vi "I(V) at various fields_K6221-K2182A_PK.vi"() -> ()   [LabVIEW 2016]
uses:
  Labview Drivers/Keithley 622x LV 2009/Keithley 622x.lvlib
panel:
  in  "Numeric Average":i32=50
  out "Iset (A)":dbl=-4.3999999999999985e-06
  out "data":dbl[](array[numeric])=[-1.0767123e-06, -4.299999999999999e-06, 0.25039820930232565]
  out "I vs V":cluster{dbl, "Field Reading":dbl}[](graph)=[{-2.65213861e-07, "Field Reading"=0.0}, {-2.06331562e-07, "Field Reading"=1e-07}, {-2.45753416e-07, "Field Reading"=2e-07}, {-2.41658661e-07, "Field Reading"=3e-07}, {-2.45242211e-07, "Field Reading"=4e-07}, {-2.44727893e-07, "Field Reading"=5e-07}, {-1.955806e-07, "Field Reading"=6e-07}, {-2.17089385e-07, "Field Reading"=7e-07}, {-2.81598074e-07, "Field Reading"=8e-07}, {-2.74937155e-07, "Field Reading"=9e-07}, {-2.57527922e-07, "Field Reading"=1e-06}, {-1.97112335e-07, "Field Reading"=1.1e-06}, {-1.8175889e-07, "Field Reading"=1.2e-06}, {-2.14527365e-07, "Field Reading"=1.2999999999999998e-06}, {-1.61276589e-07, "Field Reading"=1.3999999999999997e-06}, {-5.88852258e-08, "Field Reading"=1.4999999999999996e-06}, {4.14620688e-08, "Field Reading"=1.5999999999999995e-06}, {4.55608442e-08, "Field Reading"=1.6999999999999994e-06}, {1.10074806e-07, "Field Reading"=1.7999999999999993e-06}, {9.16432587e-08, "Field Reading"=1.8999999999999992e-06}, {2.22710882e-07, "Field Reading"=1.999999999999999e-06}, {2.90806804e-07, "Field Reading"=2.099999999999999e-06}, {2.74933923e-07, "Field Reading"=2.199999999999999e-06}, {2.81079697e-07, "Field Reading"=2.2999999999999987e-06}, {3.16914884e-07, "Field Reading"=2.3999999999999986e-06}, {2.95409204e-07, "Field Reading"=2.4999999999999985e-06}, {3.58898183e-07, "Field Reading"=2.5999999999999984e-06}, {3.56848457e-07, "Field Reading"=2.6999999999999983e-06}, {4.40815949e-07, "Field Reading"=2.799999999999998e-06}, {4.45430022e-07, "Field Reading"=2.899999999999998e-06}, {4.50042171e-07, "Field Reading"=2.999999999999998e-06}, {5.23763566e-07, "Field Reading"=3.099999999999998e-06}, {5.54477469e-07, "Field Reading"=3.1999999999999977e-06}, {5.89806137e-07, "Field Reading"=3.2999999999999976e-06}, {6.03627656e-07, "Field Reading"=3.3999999999999975e-06}, {6.54317135e-07, "Field Reading"=3.4999999999999974e-06}, {7.12174301e-07, "Field Reading"=3.5999999999999973e-06}, {7.36747564e-07, "Field Reading"=3.699999999999997e-06}, {8.03819501e-07, "Field Reading"=3.799999999999997e-06}, {8.68836656e-07, "Field Reading"=3.899999999999997e-06}, {9.59970204e-07, "Field Reading"=3.999999999999997e-06}, {9.96323249e-07, "Field Reading"=4.099999999999997e-06}, {1.07823925e-06, "Field Reading"=4.199999999999997e-06}, {1.11458965e-06, "Field Reading"=4.299999999999997e-06}, {1.11817613e-06, "Field Reading"=4.399999999999997e-06}, {1.23695717e-06, "Field Reading"=4.499999999999997e-06}, {1.24360737e-06, "Field Reading"=4.599999999999997e-06}, {1.27996158e-06, "Field Reading"=4.6999999999999965e-06}, {1.30914358e-06, "Field Reading"=4.799999999999996e-06}, {1.29941092e-06, "Field Reading"=4.899999999999996e-06}, {1.45659309e-06, "Field Reading"=4.999999999999996e-06}, {1.47759059e-06, "Field Reading"=5.099999999999996e-06}, {1.56462638e-06, "Field Reading"=5.199999999999996e-06}, {1.56923247e-06, "Field Reading"=5.299999999999996e-06}, {1.5958572e-06, "Field Reading"=5.399999999999996e-06}, {1.62196573e-06, "Field Reading"=5.499999999999996e-06}, {1.65985372e-06, "Field Reading"=5.5999999999999955e-06}, {1.66548618e-06, "Field Reading"=5.699999999999995e-06}, {1.73869841e-06, "Field Reading"=5.799999999999995e-06}, {1.75918207e-06, "Field Reading"=5.899999999999995e-06}, {1.82420779e-06, "Field Reading"=5.999999999999995e-06}, {1.87539735e-06, "Field Reading"=6.099999999999995e-06}, {2.02541342e-06, "Field Reading"=6.199999999999995e-06}, {2.05920615e-06, "Field Reading"=6.299999999999995e-06}, {2.0607414e-06, "Field Reading"=6.399999999999995e-06}, {2.09299708e-06, "Field Reading"=6.4999999999999945e-06}, {2.14470835e-06, "Field Reading"=6.599999999999994e-06}, {2.22560209e-06, "Field Reading"=6.699999999999994e-06}, {2.29164603e-06, "Field Reading"=6.799999999999994e-06}, {2.29522927e-06, "Field Reading"=6.899999999999994e-06}, {2.34898799e-06, "Field Reading"=6.999999999999994e-06}, {2.35974308e-06, "Field Reading"=7.099999999999994e-06}, {2.33516555e-06, "Field Reading"=7.199999999999994e-06}, {2.38277613e-06, "Field Reading"=7.299999999999994e-06}, {2.52971809e-06, "Field Reading"=7.3999999999999935e-06}, {2.52562488e-06, "Field Reading"=7.499999999999993e-06}, {2.53073687e-06, "Field Reading"=7.599999999999993e-06}, {2.67562896e-06, "Field Reading"=7.699999999999994e-06}, {2.75038341e-06, "Field Reading"=7.799999999999995e-06}, {2.77444721e-06, "Field Reading"=7.899999999999996e-06}, {2.86045666e-06, "Field Reading"=7.999999999999996e-06}, {2.95312204e-06, "Field Reading"=8.099999999999997e-06}, {2.99612267e-06, "Field Reading"=8.199999999999998e-06}, {2.98793425e-06, "Field Reading"=8.299999999999998e-06}, {3.08214364e-06, "Field Reading"=8.4e-06}, {3.07036496e-06, "Field Reading"=8.5e-06}, {3.17481336e-06, "Field Reading"=8.6e-06}, {3.13692748e-06, "Field Reading"=8.700000000000001e-06}, {3.13795104e-06, "Field Reading"=8.800000000000002e-06}, {3.21679593e-06, "Field Reading"=8.900000000000003e-06}, {3.24444364e-06, "Field Reading"=9.000000000000004e-06}, {3.34223395e-06, "Field Reading"=9.100000000000004e-06}, {3.37244308e-06, "Field Reading"=9.200000000000005e-06}, {3.49890549e-06, "Field Reading"=9.300000000000006e-06}, {3.5705844e-06, "Field Reading"=9.400000000000007e-06}, {3.56136e-06, "Field Reading"=9.500000000000007e-06}, {3.64941777e-06, "Field Reading"=9.600000000000008e-06}, {3.65403077e-06, "Field Reading"=9.700000000000009e-06}, {3.70881304e-06, "Field Reading"=9.80000000000001e-06}, {3.74413912e-06, "Field Reading"=9.90000000000001e-06}, {3.78202672e-06, "Field Reading"=1.0000000000000011e-05}, {3.77588359e-06, "Field Reading"=1.0100000000000012e-05}, {3.79482737e-06, "Field Reading"=1.0200000000000012e-05}, {3.84807257e-06, "Field Reading"=1.0300000000000013e-05}, {3.96326851e-06, "Field Reading"=1.0400000000000014e-05}, {4.02675375e-06, "Field Reading"=1.0500000000000015e-05}, {4.01548692e-06, "Field Reading"=1.0600000000000015e-05}, {4.03188336e-06, "Field Reading"=1.0700000000000016e-05}, {4.11892625e-06, "Field Reading"=1.0800000000000017e-05}, {4.16499723e-06, "Field Reading"=1.0900000000000018e-05}, {4.13786622e-06, "Field Reading"=1.1000000000000018e-05}, {4.15936464e-06, "Field Reading"=1.1100000000000019e-05}, {4.15372248e-06, "Field Reading"=1.120000000000002e-05}, {4.1921208e-06, "Field Reading"=1.130000000000002e-05}, {4.20441259e-06, "Field Reading"=1.1400000000000021e-05}, {4.22285166e-06, "Field Reading"=1.1500000000000022e-05}, {4.41023425e-06, "Field Reading"=1.1600000000000023e-05}, {4.43121181e-06, "Field Reading"=1.1700000000000024e-05}, {4.48548487e-06, "Field Reading"=1.1800000000000024e-05}, {4.51827063e-06, "Field Reading"=1.1900000000000025e-05}, {4.56332253e-06, "Field Reading"=1.2000000000000026e-05}, {4.56996768e-06, "Field Reading"=1.2100000000000026e-05}, {4.61196138e-06, "Field Reading"=1.2200000000000027e-05}, {4.66060156e-06, "Field Reading"=1.2300000000000028e-05}, {4.71282017e-06, "Field Reading"=1.2400000000000029e-05}, {4.72562207e-06, "Field Reading"=1.250000000000003e-05}, {4.80549203e-06, "Field Reading"=1.260000000000003e-05}, {4.84132842e-06, "Field Reading"=1.2700000000000031e-05}, {4.81931379e-06, "Field Reading"=1.2800000000000032e-05}, {4.91812376e-06, "Field Reading"=1.2900000000000032e-05}, {4.97443564e-06, "Field Reading"=1.3000000000000033e-05}, {5.06864178e-06, "Field Reading"=1.3100000000000034e-05}, {5.15414621e-06, "Field Reading"=1.3200000000000035e-05}, {5.14594912e-06, "Field Reading"=1.3300000000000035e-05}, {5.15516684e-06, "Field Reading"=1.3400000000000036e-05}, {5.24221524e-06, "Field Reading"=1.3500000000000037e-05}, {5.29853469e-06, "Field Reading"=1.3600000000000038e-05}, {5.35638168e-06, "Field Reading"=1.3700000000000038e-05}, {5.37020179e-06, "Field Reading"=1.3800000000000039e-05}, {5.3492118e-06, "Field Reading"=1.390000000000004e-05}, {5.39375972e-06, "Field Reading"=1.400000000000004e-05}, {5.47056068e-06, "Field Reading"=1.4100000000000041e-05}, {5.50895206e-06, "Field Reading"=1.4200000000000042e-05}, {5.5514459e-06, "Field Reading"=1.4300000000000043e-05}, {5.55707986e-06, "Field Reading"=1.4400000000000043e-05}, {5.60366331e-06, "Field Reading"=1.4500000000000044e-05}, {5.64206701e-06, "Field Reading"=1.4600000000000045e-05}, {5.75061982e-06, "Field Reading"=1.4700000000000046e-05}, {5.78440485e-06, "Field Reading"=1.4800000000000046e-05}, {5.84225116e-06, "Field Reading"=1.4900000000000047e-05}, {5.85863506e-06, "Field Reading"=1.5000000000000048e-05}, {5.91290279e-06, "Field Reading"=1.5100000000000049e-05}, {5.90009794e-06, "Field Reading"=1.520000000000005e-05}, {5.99225908e-06, "Field Reading"=1.530000000000005e-05}, {6.0357811e-06, "Field Reading"=1.540000000000005e-05}, {6.09005686e-06, "Field Reading"=1.5500000000000048e-05}, {6.16276569e-06, "Field Reading"=1.5600000000000047e-05}, {6.223172e-06, "Field Reading"=1.5700000000000046e-05}, {6.27077906e-06, "Field Reading"=1.5800000000000045e-05}, {6.31429835e-06, "Field Reading"=1.5900000000000044e-05}, {6.34911719e-06, "Field Reading"=1.6000000000000043e-05}, {6.38342782e-06, "Field Reading"=1.6100000000000042e-05}, {6.40851838e-06, "Field Reading"=1.620000000000004e-05}, {6.46738862e-06, "Field Reading"=1.630000000000004e-05}, {6.49911838e-06, "Field Reading"=1.640000000000004e-05}, {6.55799613e-06, "Field Reading"=1.650000000000004e-05}, {6.62046237e-06, "Field Reading"=1.6600000000000038e-05}, {6.63786331e-06, "Field Reading"=1.6700000000000037e-05}, {6.73360462e-06, "Field Reading"=1.6800000000000036e-05}, {6.76740248e-06, "Field Reading"=1.6900000000000035e-05}, {6.79761286e-06, "Field Reading"=1.7000000000000034e-05}, {6.87696878e-06, "Field Reading"=1.7100000000000033e-05}, {6.92663472e-06, "Field Reading"=1.7200000000000032e-05}, {6.96504415e-06, "Field Reading"=1.730000000000003e-05}, {7.05310834e-06, "Field Reading"=1.740000000000003e-05}, {7.1360323e-06, "Field Reading"=1.750000000000003e-05}, {7.18210114e-06, "Field Reading"=1.7600000000000028e-05}, {7.20208147e-06, "Field Reading"=1.7700000000000027e-05}, {7.28861423e-06, "Field Reading"=1.7800000000000026e-05}, {7.33519871e-06, "Field Reading"=1.7900000000000025e-05}, {7.44937016e-06, "Field Reading"=1.8000000000000024e-05}, {7.48215567e-06, "Field Reading"=1.8100000000000023e-05}, {7.55229248e-06, "Field Reading"=1.8200000000000022e-05}, {7.5732755e-06, "Field Reading"=1.830000000000002e-05}, {7.68847322e-06, "Field Reading"=1.840000000000002e-05}, {7.65775525e-06, "Field Reading"=1.850000000000002e-05}, {7.67208615e-06, "Field Reading"=1.860000000000002e-05}, {7.7637263e-06, "Field Reading"=1.8700000000000017e-05}, {7.84923772e-06, "Field Reading"=1.8800000000000017e-05}, {7.85384559e-06, "Field Reading"=1.8900000000000016e-05}, {7.90913653e-06, "Field Reading"=1.9000000000000015e-05}, {7.93422015e-06, "Field Reading"=1.9100000000000014e-05}, {8.02791857e-06, "Field Reading"=1.9200000000000013e-05}, {8.06375894e-06, "Field Reading"=1.9300000000000012e-05}, {8.08936091e-06, "Field Reading"=1.940000000000001e-05}, {8.13646665e-06, "Field Reading"=1.950000000000001e-05}, {8.17230556e-06, "Field Reading"=1.960000000000001e-05}, {8.25165814e-06, "Field Reading"=1.9700000000000008e-05}, {8.28083444e-06, "Field Reading"=1.9800000000000007e-05}, {8.32742883e-06, "Field Reading"=1.9900000000000006e-05}, {8.40371126e-06, "Field Reading"=2e-05}, {8.32588703e-06, "Field Reading"=1.9900000000000003e-05}, {8.27059152e-06, "Field Reading"=1.9800000000000004e-05}, {8.24550498e-06, "Field Reading"=1.9700000000000005e-05}, {8.18766651e-06, "Field Reading"=1.9600000000000005e-05}, {8.16002117e-06, "Field Reading"=1.9500000000000006e-05}, {8.11034423e-06, "Field Reading"=1.9400000000000007e-05}, {8.06631431e-06, "Field Reading"=1.930000000000001e-05}, {7.96853626e-06, "Field Reading"=1.920000000000001e-05}, {7.96494837e-06, "Field Reading"=1.910000000000001e-05}, {7.88456389e-06, "Field Reading"=1.900000000000001e-05}, {7.84667228e-06, "Field Reading"=1.8900000000000012e-05}, {7.76577688e-06, "Field Reading"=1.8800000000000013e-05}, {7.72174608e-06, "Field Reading"=1.8700000000000014e-05}, {7.70996248e-06, "Field Reading"=1.8600000000000015e-05}, {7.64032909e-06, "Field Reading"=1.8500000000000016e-05}, {7.58196852e-06, "Field Reading"=1.8400000000000017e-05}, {7.52616124e-06, "Field Reading"=1.8300000000000018e-05}, {7.43451656e-06, "Field Reading"=1.820000000000002e-05}, {7.419165e-06, "Field Reading"=1.810000000000002e-05}, {7.41302153e-06, "Field Reading"=1.800000000000002e-05}, {7.40278217e-06, "Field Reading"=1.7900000000000022e-05}, {7.34748378e-06, "Field Reading"=1.7800000000000023e-05}, {7.26146266e-06, "Field Reading"=1.7700000000000024e-05}, {7.22614421e-06, "Field Reading"=1.7600000000000025e-05}, {7.15294258e-06, "Field Reading"=1.7500000000000026e-05}, {7.13912167e-06, "Field Reading"=1.7400000000000027e-05}, {7.05105581e-06, "Field Reading"=1.7300000000000027e-05}, {7.06896784e-06, "Field Reading"=1.720000000000003e-05}, {6.98551895e-06, "Field Reading"=1.710000000000003e-05}, {6.92254427e-06, "Field Reading"=1.700000000000003e-05}, {6.86724585e-06, "Field Reading"=1.690000000000003e-05}, {6.85240011e-06, "Field Reading"=1.6800000000000032e-05}, {6.78225464e-06, "Field Reading"=1.6700000000000033e-05}, {6.77713724e-06, "Field Reading"=1.6600000000000034e-05}, {6.69368315e-06, "Field Reading"=1.6500000000000035e-05}, {6.63224313e-06, "Field Reading"=1.6400000000000036e-05}, {6.64145914e-06, "Field Reading"=1.6300000000000037e-05}, {6.55391401e-06, "Field Reading"=1.6200000000000038e-05}, {6.54776972e-06, "Field Reading"=1.610000000000004e-05}, {6.44434302e-06, "Field Reading"=1.600000000000004e-05}, {6.37830276e-06, "Field Reading"=1.590000000000004e-05}, {6.32249712e-06, "Field Reading"=1.5800000000000042e-05}, {6.30507964e-06, "Field Reading"=1.5700000000000043e-05}, {6.27589889e-06, "Field Reading"=1.5600000000000044e-05}, {6.19193872e-06, "Field Reading"=1.5500000000000045e-05}, {6.14893632e-06, "Field Reading"=1.5400000000000046e-05}, {6.10695312e-06, "Field Reading"=1.5300000000000047e-05}, {6.07315478e-06, "Field Reading"=1.5200000000000046e-05}, {6.01376066e-06, "Field Reading"=1.5100000000000045e-05}, {6.01273927e-06, "Field Reading"=1.5000000000000044e-05}, {5.94362298e-06, "Field Reading"=1.4900000000000044e-05}, {5.89037156e-06, "Field Reading"=1.4800000000000043e-05}, {5.87757219e-06, "Field Reading"=1.4700000000000042e-05}, {5.83406487e-06, "Field Reading"=1.4600000000000041e-05}, {5.7818526e-06, "Field Reading"=1.450000000000004e-05}, {5.79054303e-06, "Field Reading"=1.440000000000004e-05}, {5.72397236e-06, "Field Reading"=1.430000000000004e-05}, {5.69632955e-06, "Field Reading"=1.4200000000000039e-05}, {5.62875043e-06, "Field Reading"=1.4100000000000038e-05}, {5.61902647e-06, "Field Reading"=1.4000000000000037e-05}, {5.53097021e-06, "Field Reading"=1.3900000000000036e-05}, {5.58626586e-06, "Field Reading"=1.3800000000000036e-05}, {5.5396681e-06, "Field Reading"=1.3700000000000035e-05}, {5.49102684e-06, "Field Reading"=1.3600000000000034e-05}, {5.46030697e-06, "Field Reading"=1.3500000000000033e-05}, {5.39784099e-06, "Field Reading"=1.3400000000000033e-05}, {5.28981952e-06, "Field Reading"=1.3300000000000032e-05}, {5.3456268e-06, "Field Reading"=1.3200000000000031e-05}, {5.23811359e-06, "Field Reading"=1.310000000000003e-05}, {5.28317073e-06, "Field Reading"=1.300000000000003e-05}, {5.23554661e-06, "Field Reading"=1.2900000000000029e-05}, {5.18742312e-06, "Field Reading"=1.2800000000000028e-05}, {5.16080263e-06, "Field Reading"=1.2700000000000027e-05}, {5.08911473e-06, "Field Reading"=1.2600000000000027e-05}, {5.02306725e-06, "Field Reading"=1.2500000000000026e-05}, {4.95087495e-06, "Field Reading"=1.2400000000000025e-05}, {4.89097002e-06, "Field Reading"=1.2300000000000025e-05}, {4.85103666e-06, "Field Reading"=1.2200000000000024e-05}, {4.81161312e-06, "Field Reading"=1.2100000000000023e-05}, {4.8223712e-06, "Field Reading"=1.2000000000000022e-05}, {4.71997748e-06, "Field Reading"=1.1900000000000022e-05}, {4.70513009e-06, "Field Reading"=1.1800000000000021e-05}, {4.61860758e-06, "Field Reading"=1.170000000000002e-05}, {4.50494221e-06, "Field Reading"=1.160000000000002e-05}, {4.50442328e-06, "Field Reading"=1.1500000000000019e-05}, {4.48907395e-06, "Field Reading"=1.1400000000000018e-05}, {4.48549552e-06, "Field Reading"=1.1300000000000017e-05}, {4.43275985e-06, "Field Reading"=1.1200000000000016e-05}, {4.37336829e-06, "Field Reading"=1.1100000000000016e-05}, {4.35544798e-06, "Field Reading"=1.1000000000000015e-05}, {4.23615778e-06, "Field Reading"=1.0900000000000014e-05}, {4.18496019e-06, "Field Reading"=1.0800000000000013e-05}, {4.13529928e-06, "Field Reading"=1.0700000000000013e-05}, {4.0963864e-06, "Field Reading"=1.0600000000000012e-05}, {4.10252432e-06, "Field Reading"=1.0500000000000011e-05}, {4.14245452e-06, "Field Reading"=1.040000000000001e-05}, {4.0723185e-06, "Field Reading"=1.030000000000001e-05}, {3.99655577e-06, "Field Reading"=1.0200000000000009e-05}, {3.91820595e-06, "Field Reading"=1.0100000000000008e-05}, {3.90693848e-06, "Field Reading"=1.0000000000000008e-05}, {3.90182893e-06, "Field Reading"=9.900000000000007e-06}, {3.89824771e-06, "Field Reading"=9.800000000000006e-06}, {3.89568225e-06, "Field Reading"=9.700000000000005e-06}, {3.82297919e-06, "Field Reading"=9.600000000000005e-06}, {3.79072008e-06, "Field Reading"=9.500000000000004e-06}, {3.75283128e-06, "Field Reading"=9.400000000000003e-06}, {3.74925146e-06, "Field Reading"=9.300000000000002e-06}, {3.69600662e-06, "Field Reading"=9.200000000000002e-06}, {3.68985764e-06, "Field Reading"=9.100000000000001e-06}, {3.53830951e-06, "Field Reading"=9e-06}, {3.48967903e-06, "Field Reading"=8.9e-06}, {3.4169754e-06, "Field Reading"=8.799999999999999e-06}, {3.35195893e-06, "Field Reading"=8.699999999999998e-06}, {3.26798993e-06, "Field Reading"=8.599999999999997e-06}, {3.32840376e-06, "Field Reading"=8.499999999999997e-06}, {3.28130617e-06, "Field Reading"=8.399999999999996e-06}, {3.22038204e-06, "Field Reading"=8.299999999999995e-06}, {3.19170899e-06, "Field Reading"=8.199999999999994e-06}, {3.14817946e-06, "Field Reading"=8.099999999999994e-06}, {3.06473437e-06, "Field Reading"=7.999999999999993e-06}, {3.0155901e-06, "Field Reading"=7.899999999999992e-06}, {2.89219787e-06, "Field Reading"=7.799999999999991e-06}, {2.84355222e-06, "Field Reading"=7.69999999999999e-06}, {2.79798017e-06, "Field Reading"=7.599999999999991e-06}, {2.73245105e-06, "Field Reading"=7.499999999999991e-06}, {2.68023355e-06, "Field Reading"=7.399999999999991e-06}, {2.76420187e-06, "Field Reading"=7.299999999999991e-06}, {2.74935814e-06, "Field Reading"=7.199999999999991e-06}, {2.68791939e-06, "Field Reading"=7.099999999999991e-06}, {2.63261821e-06, "Field Reading"=6.9999999999999914e-06}, {2.60291933e-06, "Field Reading"=6.8999999999999915e-06}, {2.51843848e-06, "Field Reading"=6.799999999999992e-06}, {2.5061508e-06, "Field Reading"=6.699999999999992e-06}, {2.33208474e-06, "Field Reading"=6.599999999999992e-06}, {2.3167298e-06, "Field Reading"=6.499999999999992e-06}, {2.30443977e-06, "Field Reading"=6.399999999999992e-06}, {2.24402212e-06, "Field Reading"=6.299999999999992e-06}, {2.26142112e-06, "Field Reading"=6.199999999999992e-06}, {2.24708744e-06, "Field Reading"=6.099999999999992e-06}, {2.18258492e-06, "Field Reading"=5.9999999999999925e-06}, {2.06226311e-06, "Field Reading"=5.899999999999993e-06}, {1.97317707e-06, "Field Reading"=5.799999999999993e-06}, {1.89791536e-06, "Field Reading"=5.699999999999993e-06}, {1.8943317e-06, "Field Reading"=5.599999999999993e-06}, {1.91123261e-06, "Field Reading"=5.499999999999993e-06}, {1.79142144e-06, "Field Reading"=5.399999999999993e-06}, {1.82674468e-06, "Field Reading"=5.299999999999993e-06}, {1.75353415e-06, "Field Reading"=5.199999999999993e-06}, {1.65932968e-06, "Field Reading"=5.0999999999999935e-06}, {1.65933232e-06, "Field Reading"=4.999999999999994e-06}, {1.54669792e-06, "Field Reading"=4.899999999999994e-06}, {1.44584143e-06, "Field Reading"=4.799999999999994e-06}, {1.52673386e-06, "Field Reading"=4.699999999999994e-06}, {1.4320141e-06, "Field Reading"=4.599999999999994e-06}, {1.40795279e-06, "Field Reading"=4.499999999999994e-06}, {1.32296227e-06, "Field Reading"=4.399999999999994e-06}, {1.08181445e-06, "Field Reading"=4.299999999999994e-06}, {1.07105849e-06, "Field Reading"=4.1999999999999945e-06}, {1.07361536e-06, "Field Reading"=4.099999999999995e-06}, {1.06030613e-06, "Field Reading"=3.999999999999995e-06}, {9.90675451e-07, "Field Reading"=3.899999999999995e-06}, {9.98353274e-07, "Field Reading"=3.799999999999995e-06}, {9.51769766e-07, "Field Reading"=3.699999999999995e-06}, {9.19007087e-07, "Field Reading"=3.599999999999995e-06}, {8.96477356e-07, "Field Reading"=3.4999999999999953e-06}, {8.37598555e-07, "Field Reading"=3.3999999999999954e-06}, {7.43906148e-07, "Field Reading"=3.2999999999999955e-06}, {7.07042824e-07, "Field Reading"=3.1999999999999956e-06}, {7.8384287e-07, "Field Reading"=3.0999999999999957e-06}, {6.97316697e-07, "Field Reading"=2.999999999999996e-06}, {6.99871857e-07, "Field Reading"=2.899999999999996e-06}, {6.61988855e-07, "Field Reading"=2.799999999999996e-06}, {6.67112949e-07, "Field Reading"=2.699999999999996e-06}, {5.21710306e-07, "Field Reading"=2.5999999999999963e-06}, {5.11980802e-07, "Field Reading"=2.4999999999999964e-06}, {5.26306067e-07, "Field Reading"=2.3999999999999965e-06}, {5.57538796e-07, "Field Reading"=2.2999999999999966e-06}, {5.49862592e-07, "Field Reading"=2.1999999999999967e-06}, {4.38246539e-07, "Field Reading"=2.099999999999997e-06}, {4.53099149e-07, "Field Reading"=1.999999999999997e-06}, {3.79374306e-07, "Field Reading"=1.899999999999997e-06}, {3.25102595e-07, "Field Reading"=1.7999999999999972e-06}, {2.04792301e-07, "Field Reading"=1.6999999999999973e-06}, {2.36019239e-07, "Field Reading"=1.5999999999999974e-06}, {2.33452923e-07, "Field Reading"=1.4999999999999975e-06}, {2.2372704e-07, "Field Reading"=1.3999999999999976e-06}, {2.67761542e-07, "Field Reading"=1.2999999999999977e-06}, {2.54450874e-07, "Field Reading"=1.1999999999999978e-06}, {1.63316468e-07, "Field Reading"=1.099999999999998e-06}, {7.72994096e-08, "Field Reading"=9.99999999999998e-07}, {8.85529671e-08, "Field Reading"=8.999999999999981e-07}, {7.06354729e-08, "Field Reading"=7.999999999999981e-07}, {1.87884609e-07, "Field Reading"=6.999999999999981e-07}, {1.58696118e-07, "Field Reading"=5.999999999999981e-07}, {1.73034013e-07, "Field Reading"=4.999999999999981e-07}, {1.02383086e-07, "Field Reading"=3.999999999999981e-07}, {6.60310964e-08, "Field Reading"=2.999999999999981e-07}, {1.43341752e-07, "Field Reading"=1.9999999999999809e-07}, {2.34987166e-07, "Field Reading"=9.999999999999809e-08}, {1.56651714e-07, "Field Reading"=-1.9058241313221758e-21}, {1.5204492e-07, "Field Reading"=-1.000000000000019e-07}, {2.03758966e-07, "Field Reading"=-2.000000000000019e-07}, {2.2474776e-07, "Field Reading"=-3.000000000000019e-07}, {1.65354644e-07, "Field Reading"=-4.000000000000019e-07}, {1.18764208e-07, "Field Reading"=-5.000000000000019e-07}, {7.88302354e-08, "Field Reading"=-6.000000000000019e-07}, {1.93518827e-07, "Field Reading"=-7.000000000000019e-07}, {1.5665572e-07, "Field Reading"=-8.000000000000019e-07}, {2.47273023e-07, "Field Reading"=-9.000000000000019e-07}, {2.08356789e-07, "Field Reading"=-1.0000000000000019e-06}, {2.10917939e-07, "Field Reading"=-1.1000000000000018e-06}, {1.69965974e-07, "Field Reading"=-1.2000000000000016e-06}, {1.11596254e-07, "Field Reading"=-1.3000000000000015e-06}, {9.20117195e-09, "Field Reading"=-1.4000000000000014e-06}, {-7.42491073e-08, "Field Reading"=-1.5000000000000013e-06}, {-7.5273293e-08, "Field Reading"=-1.6000000000000012e-06}, {-6.65732606e-08, "Field Reading"=-1.700000000000001e-06}, {-1.58906482e-08, "Field Reading"=-1.800000000000001e-06}, {-1.34670081e-07, "Field Reading"=-1.9000000000000009e-06}, {-2.32454805e-07, "Field Reading"=-2.0000000000000008e-06}, {-2.82111171e-07, "Field Reading"=-2.1000000000000006e-06}, {-3.47645977e-07, "Field Reading"=-2.2000000000000005e-06}, {-3.37922223e-07, "Field Reading"=-2.3000000000000004e-06}, {-3.85029026e-07, "Field Reading"=-2.4000000000000003e-06}, {-2.86727063e-07, "Field Reading"=-2.5e-06}, {-2.61119956e-07, "Field Reading"=-2.6e-06}, {-2.56507099e-07, "Field Reading"=-2.7e-06}, {-3.87066578e-07, "Field Reading"=-2.8e-06}, {-5.12512258e-07, "Field Reading"=-2.8999999999999998e-06}, {-5.18652063e-07, "Field Reading"=-2.9999999999999997e-06}, {-5.77529798e-07, "Field Reading"=-3.0999999999999995e-06}, {-6.54844775e-07, "Field Reading"=-3.1999999999999994e-06}, {-6.1951305e-07, "Field Reading"=-3.2999999999999993e-06}, {-6.40503708e-07, "Field Reading"=-3.399999999999999e-06}, {-6.31290379e-07, "Field Reading"=-3.499999999999999e-06}, {-6.56374953e-07, "Field Reading"=-3.599999999999999e-06}, {-6.85558188e-07, "Field Reading"=-3.699999999999999e-06}, {-7.71570974e-07, "Field Reading"=-3.7999999999999988e-06}, {-9.11853044e-07, "Field Reading"=-3.899999999999999e-06}, {-9.0314763e-07, "Field Reading"=-3.999999999999999e-06}, {-9.40523971e-07, "Field Reading"=-4.099999999999999e-06}, {-1.02704958e-06, "Field Reading"=-4.199999999999999e-06}, {-1.0767123e-06, "Field Reading"=-4.299999999999999e-06}]
  in  "wait (ms)":u32=1000
  in  "Set Compliance voltage (V)":dbl=2.0 min=0.0 step=0.1 format="%_3f"
  in  "Nanovoltmeter 2182a VISA":refnum<visa-resource-name>="COM1"
  in  "Current source K6221 VISA":refnum<visa-resource-name>="COM1"
  out "Time (s)":dbl format="%#_13g"
  in  "Field ramp rate (T/min)":string="0.05"
  in  "Magnetic field stabilization time (s)":dbl=200.0 format="%#_13g"
  in  "Step 2":dbl[](array[numeric])=[0.25] min=-3000.0 max=3000.0 format="%.1e"
  in  "To 2":dbl[](array[numeric])=[6.0] min=-3000.0 max=3000.0 format="%.1e"
  in  "From 2":dbl[](array[numeric])=[8.5] min=-3000.0 max=3000.0 format="%.1e"
  out "Magnetic Field (T)":dbl format="%#_13g"
  in  "Magnet IP Address":string="169.254.46.132"
  out "Vmeas (V)":dbl=nan
  in  "Folder":path=path "D:/Pranava/Data/NbO/27-05-2020"
  in  "Step":dbl[](array[numeric])=[0.001, 0.001, 0.001] min=-3000.0 max=3000.0 format="%.1e"
  in  "To":dbl[](array[numeric])=[0.5, -0.5, 0.0] min=-3000.0 max=3000.0 format="%.1e"
  in  "From":dbl[](array[numeric])=[0.0, 0.5, -0.5] min=-3000.0 max=3000.0 format="%.1e"
  in  "file name":string="001_IV_(Nb)STO_7mK_MFLI_MF-MD"
  out "File path":path=path "D:/Pranava/Data/001_IV_(Nb)STO_7mK_MFLI_MF-MD.dat"
  # ".dat"
  # "[Must be less than 0.05]"
  # "Configure Magnetic field sweep (T)"
  # "Set Current sweep (A)"
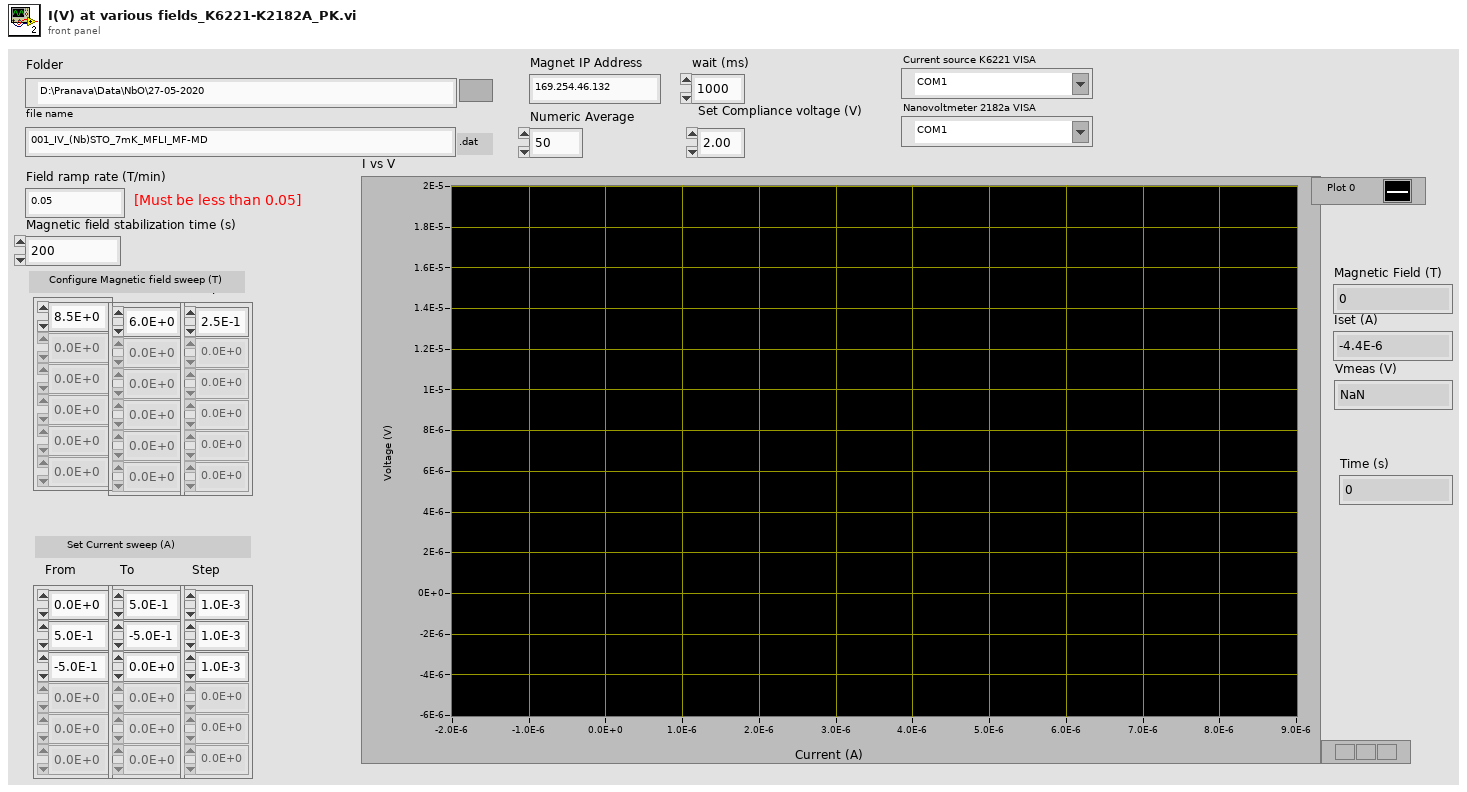
[diagram p1: front panel]
types:
  T1 = enum16{"open", "replace", "create", "open or create", "replace or create", "replace or create with confirmation"}
  T2 = typedef "Keithley 622x.lvlib/KE622x -- Current Level.ctl" = dbl
  T3 = cluster{"Average value":dbl, "Average value":dbl}
  T4 = cluster{"Average value":dbl, "Average value":dbl}[]
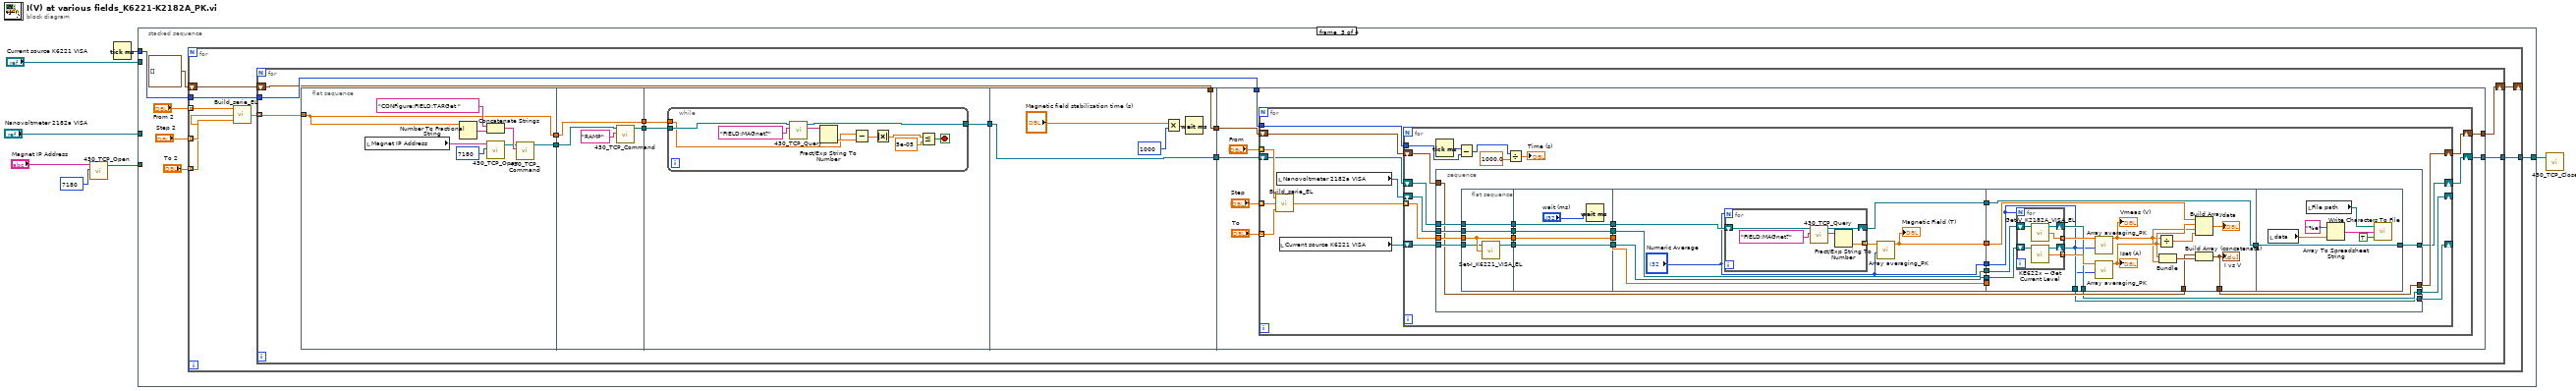
[diagram p0: block diagram]
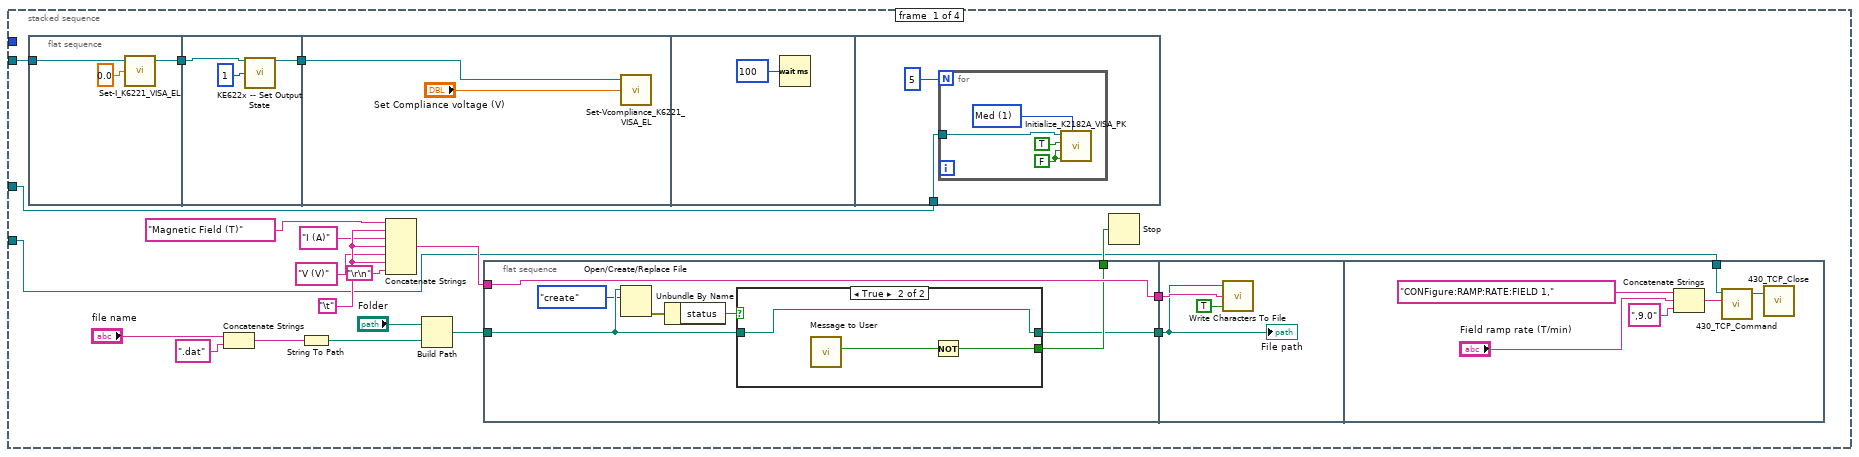
[diagram p2: hidden frame]
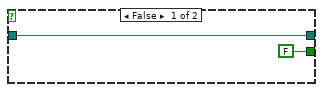
[diagram p3: hidden frame]
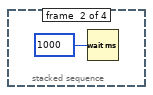
[diagram p4: hidden frame]
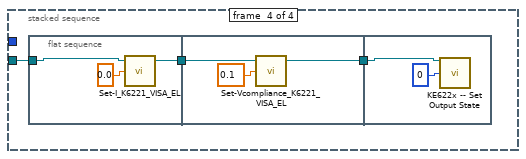
[diagram p5: hidden frame]
diagram:
  n1 = call "430_TCP_Open.vi"("IP Address"="Magnet IP Address", "TCP Port"=7180) -> ("connection ID"=w4:refnum<k5>)  [unwired: 4 in, 2 out]
  n2 = Tick Count (ms)() -> (millisecond timer value=w3:u32)
  n3 = stacked-sequence {
    tunnel: [_ _ w67 _] -> w7
    tunnel: w4 -> [w14 _ _ _]
    tunnel: w3 -> [_ _ w66 _]
    tunnel: "Current source K6221 VISA" -> [w10 _ _ w229]
    tunnel: "Nanovoltmeter 2182a VISA" -> [w9 _ _ _]
    frame #0 {
      w24 = "\t"
      n4 = flat-sequence {
        tunnel: w10 -> [w30]
        tunnel: [w28] -> w11
        tunnel: w11 -> [w33]
        tunnel: [w31] -> w8
        tunnel: w8 -> [w34]
        tunnel: w9 -> [w37]
        frame #0 {
          n5 = call "Set-I_K6221_VISA_EL.vi"("Set I (A)"=0.0, "K6221 VISA"=w30) -> ("K6221 VISA out"=w28:refnum<visa-resource-name>)  [unwired: 2 in, 1 out]
        }
        frame #1 {
          n6 = call "KE622x -- Set Output State.vi"("Resource In"=w33, "Output State"=1) -> ("Resource Out (dupl)"=w31:refnum<visa-resource-name>)  [unwired: 12 in, 1 out]
        }
        frame #2 {
          n7 = call "Set-Vcompliance_K6221_VISA_EL.vi"("Set Compliance voltage (V)"="Set Compliance voltage (V)", "K6221 VISA"=w34) -> ()  [unwired: 2 in, 2 out]
        }
        frame #3 {
          n8 = Wait (ms)(milliseconds to wait=100) -> ()  [unwired: 1 out]
        }
        frame #4 {
          n9 = for {
            N: 5 ("Numeric") -> [_]
            tunnel: w37 -> [w39]
            w41 = u16 1 items=["Slow", "Med", "Fast"] ("Rate (NPLC)")
            w42 = FALSE ("Auto range?")
            n10 = call "Initialize_K2182A_VISA_PK.vi"("VISA address"=w39, "Auto range?"=TRUE, "Analog LPass\nFilter?"=w42, "DC\nFilter?"=w42, "Rate (NPLC)"=w41) -> ()  [unwired: 2 in]
          }
        }
      }
      n11 = Concatenate Strings("file name", ".dat" ("string")) -> (w22:string)
      n12 = String To Path(string=w22) -> (path=w16:path)
      n13 = Concatenate Strings("Magnetic Field (T)", w24, "I (A)" ("string"), w24, "V (V)" ("string"), w24, "\r\n") -> (w23:string)
      n14 = Build Path(base path="Folder", name or relative path=w16) -> (appended path=w15:path)
      n15 = flat-sequence {
        tunnel: w15 -> [w46]
        tunnel: w23 -> [w49]
        tunnel: [w49] -> w27
        tunnel: [w48] -> w20
        tunnel: [w47] -> w26
        tunnel: w27 -> [w56]
        tunnel: w26 -> [w55]
        tunnel: w14 -> [w58]
        frame #0 {
          n16 = Open/Create/Replace File(file path (use dialog)=w46, operation (0:open)=T1."create") -> (error out=w45:errorcluster)  [unwired: 4 in, 2 out]
          n17 = Unbundle By Name(w45) -> ("status"=w43:bool)
          n18 = case shown="True" w43 {
            tunnel: [FALSE ("Yes") w53] -> w48
            tunnel: [w50 w52] -> w47
            tunnel: w46 -> [w50 w52]
            frame False {
            }
            frame True {
              n19 = call "Message to User"() -> ("Yes"=w54:bool)  [unwired: 10 in, 1 out]
              n20 = Not(x=w54) -> (.not. x?=w53:bool)
            }
          }
        }
        frame #1 {
          n21 = call <vilib>:"Write Characters To File.vi"("append to file? (new file:F)"=TRUE, "character string"=w56, "file path (dialog if empty)"=w55) -> ()  [unwired: 2 in, 1 out]
          "File path" <- w55
        }
        frame #2 {
          n22 = Concatenate Strings("CONFigure:RAMP:RATE:FIELD 1," ("String"), "Field ramp rate (T/min)", ",9.0") -> (w59:string)
          n23 = call "430_TCP_Command.vi"("Command"=w59, "connection ID"=w58) -> ("connection ID out"=w63:refnum<k5>)  [unwired: 2 in, 2 out]
          n24 = call "430_TCP_Close.vi"("connection ID"=w63) -> ()  [unwired: 1 in, 2 out]
        }
      }
      n25 = Stop(stop? (T)=w20) -> ()
    }
    frame #1 {
      n26 = Wait (ms)(milliseconds to wait=u32 1000) -> ()  [unwired: 1 out]
    }
    frame #2 {
      n27 = for {
        tunnel: "From 2" -> [w78] mode=indexing
        tunnel: "To 2" -> [w76] mode=indexing
        tunnel: "Step 2" -> [w77] mode=indexing
        tunnel: [w74] -> w67
        tunnel: w66 -> [w73]
        shift-right: [w71] -> _
        shift-left: cluster{dbl, "Field Reading":dbl}[] [] -> [w72]
        n28 = call "Build_serie_EL.vi"("end value"=w76, "increment"=w77, "start value"=w78) -> ("output array"=w75:dbl[])
        n29 = for {
          tunnel: w75 -> [w90] mode=indexing
          tunnel: [w85] -> w74
          tunnel: w73 -> [w82]
          shift-right: [w79] -> w71
          shift-left: w72 -> [w80]
          n30 = flat-sequence {
            tunnel: w90 -> [w94]
            tunnel: [w95] -> w84
            tunnel: [w94] -> w83
            tunnel: [w100] -> w89
            tunnel: [w99] -> w88
            tunnel: w83 -> [w99]
            tunnel: w84 -> [w102]
            tunnel: w89 -> [w105]
            tunnel: w88 -> [w104]
            tunnel: [w103] -> w86
            tunnel: [w117] -> w87
            tunnel: w86 -> [w117]
            tunnel: [w116] -> w81
            tunnel: w80 -> [w116]
            tunnel: w87 -> [w125]
            tunnel: [w124] -> w85
            tunnel: w82 -> [w123]
            tunnel: w81 -> [w122]
            tunnel: [w121] -> w79
            frame #0 {
              n31 = local read "Magnet IP Address"() -> (w92:string)
              n32 = Number To Fractional String(number=w94) -> (F-format string=w96:string)  [unwired: 3 in]
              n33 = Concatenate Strings("CONFigure:FIELD:TARGet " ("String"), w96) -> (w98:string)
              n34 = call "430_TCP_Open.vi"("IP Address"=w92, "TCP Port"=7180) -> ("connection ID"=w91:refnum<k5>)  [unwired: 4 in, 2 out]
              n35 = call "430_TCP_Command.vi"("Command"=w98, "connection ID"=w91) -> ("connection ID out"=w95:refnum<k5>)  [unwired: 2 in, 2 out]
            }
            frame #1 {
              n36 = call "430_TCP_Command.vi"("Command"="RAMP", "connection ID"=w102) -> ("connection ID out"=w100:refnum<k5>)  [unwired: 2 in, 2 out]
            }
            frame #2 {
              n37 = while {
                tunnel: w105 -> [w115]
                tunnel: w104 -> [w110]
                tunnel: [w106] -> w103
                stop <- w108 stop-if-true
                n38 = call "430_TCP_Query.vi"("Command"="FIELD:MAGnet?" ("String"), "connection ID"=w115) -> ("Response"=w114:string, "connection ID out"=w106:refnum<k5>)  [unwired: 5 in, 3 out]
                n39 = Fract/Exp String To Number(string=w114) -> (number=w111:dbl)  [unwired: 3 in, 1 out]
                n40 = Subtract(x=w110, y=w111) -> (x-y=w113:dbl)
                n41 = Absolute Value(x=w113) -> (abs(x)=w112:dbl)
                n42 = Less Or Equal?(x=w112, y=5e-05) -> (x <= y?=w108:bool)
              }
            }
            frame #3 {
              n43 = Multiply(x="Magnetic field stabilization time (s)", y=1000) -> (x*y=w119:dbl)
              n44 = Wait (ms)(milliseconds to wait=w119) -> ()  [unwired: 1 out]
            }
            frame #4 {
              n45 = for {
                tunnel: "From" -> [w136] mode=indexing
                tunnel: "To" -> [w135] mode=indexing
                tunnel: "Step" -> [w134] mode=indexing
                shift-right: [w138] -> w121
                shift-left: w122 -> [w139]
                shift-right: [w132] -> w124
                shift-left: w125 -> [w133]
                tunnel: w123 -> [w131]
                n46 = call "Build_serie_EL.vi"("end value"=w135, "increment"=w134, "start value"=w136) -> ("output array"=w137:dbl[])
                n47 = local read "Nanovoltmeter 2182a VISA"() -> (w129:refnum<visa-resource-name>)
                n48 = local read "Current source K6221 VISA"() -> (w130:refnum<visa-resource-name>)
                n49 = for {
                  tunnel: w137 -> [w153] mode=indexing
                  shift-right: [w151] -> w138
                  shift-left: w139 -> [w152]
                  shift-right: [w140] -> _
                  shift-left: w130 -> [w150]
                  shift-right: [w141] -> _
                  shift-left: w129 -> [w149]
                  shift-right: [w148] -> w132
                  shift-left: w133 -> [w147]
                  tunnel: w131 -> [w143]
                  n50 = Tick Count (ms)() -> (millisecond timer value=w144:u32)
                  n51 = stacked-sequence {
                    tunnel: w153 -> [w177]
                    tunnel: w152 -> [w165]
                    tunnel: [w164] -> w151
                    tunnel: w150 -> [w176]
                    tunnel: w149 -> [w175]
                    tunnel: [w171] -> w148
                    tunnel: w147 -> [w170]
                    tunnel: [w156] -> w141
                    tunnel: [w155] -> w140
                    frame #0 {
                      n52 = flat-sequence {
                        tunnel: [w181] -> w169
                        tunnel: [w182] -> w167
                        tunnel: w170 -> [w182]
                        tunnel: w175 -> [w178]
                        tunnel: w176 -> [w180]
                        tunnel: w177 -> [w181]
                        tunnel: [w179] -> w161
                        tunnel: [w178] -> w160
                        tunnel: w169 -> [w187]
                        tunnel: [w187] -> w168
                        tunnel: w167 -> [w186]
                        tunnel: [w186] -> w166
                        tunnel: [w184] -> w162
                        tunnel: w161 -> [w184]
                        tunnel: w160 -> [w183]
                        tunnel: [w183] -> w159
                        tunnel: w168 -> [w195]
                        tunnel: [w195] -> w174
                        tunnel: [w189] -> w173
                        tunnel: [w194] -> w172
                        tunnel: w166 -> [w193]
                        tunnel: [w192] -> w163
                        tunnel: w162 -> [w192]
                        tunnel: w159 -> [w191]
                        tunnel: [w191] -> w158
                        tunnel: ["Numeric Average"] -> w154
                        tunnel: w172 -> [w216]
                        tunnel: w173 -> [w206]
                        tunnel: w174 -> [_]
                        tunnel: w165 -> [w210]
                        tunnel: [w209] -> w164
                        tunnel: w163 -> [w208]
                        tunnel: w158 -> [w207]
                        tunnel: [w216] -> w157
                        tunnel: [w203] -> w156
                        tunnel: [w202] -> w155
                        tunnel: w154 -> [w201]
                        tunnel: [w228] -> w171
                        tunnel: w157 -> [w228]
                        frame #0 {
                          n53 = call "Set-I_K6221_VISA_EL.vi"("Set I (A)"=w181, "K6221 VISA"=w180) -> ("K6221 VISA out"=w179:refnum<visa-resource-name>)  [unwired: 2 in, 1 out]
                        }
                        frame #1 {
                          n54 = Wait (ms)(milliseconds to wait="wait (ms)") -> ()  [unwired: 1 out]
                        }
                        frame #2 {
                          n55 = for {
                            N: "Numeric Average" -> [_]
                            tunnel: [w198] -> w190 mode=indexing
                            shift-right: [w197] -> w194
                            shift-left: w193 -> [w196]
                            n56 = call "430_TCP_Query.vi"("Command"="FIELD:MAGnet?" ("String"), "connection ID"=w196) -> ("Response"=w200:string, "connection ID out"=w197:refnum<k5>)  [unwired: 5 in, 3 out]
                            n57 = Fract/Exp String To Number(string=w200) -> (number=w198:dbl)  [unwired: 3 in, 1 out]
                          }
                          n58 = call "Array averaging_PK.vi"("Number averaging"="Numeric Average", "numeric array"=w190) -> ("Average value"=w189:dbl)  [unwired: 9 in]
                          "Magnetic Field (T)" <- w189
                        }
                        frame #3 {
                          n59 = for {
                            N: w201 -> [_]
                            tunnel: [w222] -> w213 mode=indexing
                            tunnel: [w221] -> w212 mode=indexing
                            shift-right: [w219] -> w202
                            shift-left: w208 -> [w220]
                            shift-right: [w217] -> w203
                            shift-left: w207 -> [w218]
                            n60 = call "Get-V_K2182A_VISA_EL.vi"("VISA K2182A"=w218) -> ("V (V)"=w222:dbl, "VISA K2182A"=w217:refnum<visa-resource-name>)  [unwired: 2 in, 1 out]
                            n61 = call "KE622x -- Get Current Level.vi"("Resource In"=w220) -> ("Resource Out (dupl)"=w219:refnum<visa-resource-name>, "Current Level (A)"=w221:T2)  [unwired: 12 in, 1 out]
                          }
                          n62 = call "Array averaging_PK.vi"("Number averaging"=w201, "numeric array"=w213) -> ("Average value"=w204:dbl)  [unwired: 9 in]
                          "Vmeas (V)" <- w204
                          n63 = call "Array averaging_PK.vi"("Number averaging"=w201, "numeric array"=w212) -> ("Average value"=w205:dbl)  [unwired: 9 in]
                          "Iset (A)" <- w205
                          n64 = Divide(x=w204, y=w205) -> (x/y=w211:dbl)
                          n65 = Bundle("Average value"=w205, "Average value"=w204) -> (w214:T3)  [unwired: 1 in]
                          n66 = Build Array(w206, w205, w204, w211) -> (→"data":dbl[])
                          n67 = Build Array (concatenate)(w210, w214) -> (w209:T4)
                          "I vs V" <- w209
                        }
                        frame #4 {
                          n68 = local read "data"() -> (w223:dbl[])
                          n69 = local read "File path"() -> (w225:path)
                          n70 = Array To Spreadsheet String(array=w223, 3:"%e" ("format string")) -> (spreadsheet string=w226:string)  [unwired: 1 in]
                          n71 = call <vilib>:"Write Characters To File.vi"("append to file? (new file:F)"=TRUE, "character string"=w226, "file path (dialog if empty)"=w225) -> ()  [unwired: 2 in, 1 out]
                        }
                      }
                    }
                  }
                  n72 = Subtract(x=w144, y=w143) -> (x-y=w146:u32)
                  n73 = Divide(x=w146, y=1000.0) -> (x/y=→"Time (s)":dbl)
                }
              }
            }
          }
        }
      }
    }
    frame #3 {
      n74 = flat-sequence {
        tunnel: w229 -> [w234]
        tunnel: [w232] -> w231
        tunnel: w231 -> [w236]
        tunnel: [w235] -> w230
        tunnel: w230 -> [w239]
        frame #0 {
          n75 = call "Set-I_K6221_VISA_EL.vi"("Set I (A)"=0.0, "K6221 VISA"=w234) -> ("K6221 VISA out"=w232:refnum<visa-resource-name>)  [unwired: 2 in, 1 out]
        }
        frame #1 {
          n76 = call "Set-Vcompliance_K6221_VISA_EL.vi"("Set Compliance voltage (V)"=0.1, "K6221 VISA"=w236) -> ("K6221 VISA out"=w235:refnum<visa-resource-name>)  [unwired: 2 in, 1 out]
        }
        frame #2 {
          n77 = call "KE622x -- Set Output State.vi"("Resource In"=w239, "Output State"=0) -> ()  [unwired: 12 in, 2 out]
        }
      }
    }
  }
  n78 = call "430_TCP_Close.vi"("connection ID"=w7) -> ()  [unwired: 1 in, 2 out]
